vi "IF2_TagDataConversion.vi"(8 "error in (no error)":errorcluster, 10 "IF2 Data":string, 11 "TCP Network Connection in":refnum<k5>) -> (0 "error out":errorcluster, 3 "TCP Network Connection out":refnum<k5>)   [LabVIEW 2015, in "IF2_Reader.lvlib"]
uses:
  IF2_Reader.lvlib
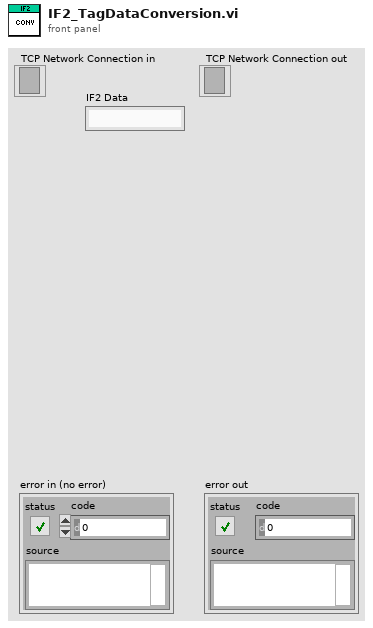
[diagram p1: front panel]
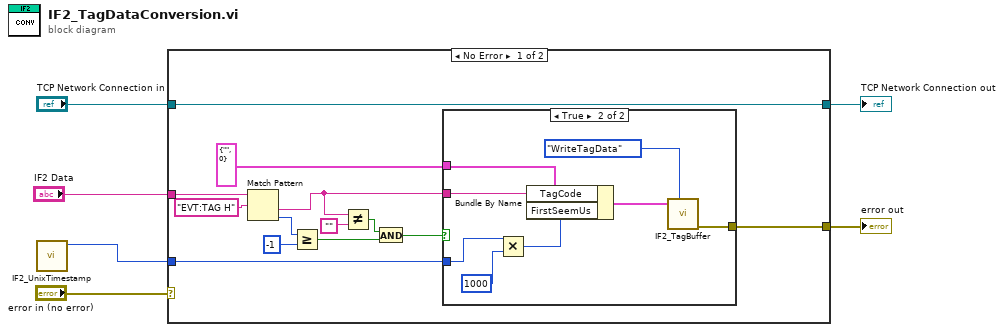
[diagram p0: block diagram]
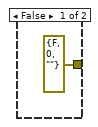
[diagram p2: hidden frame]
diagram:
  n1 = call "IF2_UnixTimestamp.vi"() -> ("unixTimeStamp"=w1:u64)  [unwired: 11 in]
  n2 = case shown="No Error" "error in (no error)" {
    selector: "error in (no error)" -> [_ w29]
    tunnel: "TCP Network Connection in" -> [w16 w30]
    tunnel: [w16 w30] -> w4
    tunnel: [w18 w29] -> w6
    tunnel: "IF2 Data" -> [w14 _]
    tunnel: w1 -> [w15 _]
    frame No Error {
      n3 = Match Pattern(string=w14, regular expression="EVT:TAG H") -> (after substring=w9:string, offset past match=w13:i32)  [unwired: 3 out]
      n4 = Greater Or Equal?(x=w13, y=-1) -> (x >= y?=w11:bool)
      n5 = Not Equal?(x=w9, y="") -> (x != y?=w7:bool)
      n6 = And(x=w7, y=w11) -> (x .and. y?=w10:bool)
      n7 = case shown="True" w10 {
        tunnel: [errorcluster {"status"=FALSE, "code"=0, "source"=""} ("error out") w23] -> w18
        tunnel: w9 -> [_ w27]
        tunnel: cluster{"TagCode":string, "FirstSeemUs":u64} {"TagCode"="", "FirstSeemUs"=0} ("TagData in") -> [_ w28]
        tunnel: w15 -> [_ w26]
        frame False {
        }
        frame True {
          n8 = Multiply(x=w26, y=u64 1000) -> (x*y=w21:u64)
          n9 = Bundle By Name(cluster=w28, "TagCode"=w27, "FirstSeemUs"=w21) -> (w24:cluster{"TagCode":string, "FirstSeemUs":u64})
          n10 = call "IF2_TagBuffer.vi"("Action"=enum16{"Init", "WriteTagData", "ReadTagData"}."WriteTagData", "TagData in"=w24) -> ("error out"=w23:errorcluster)  [unwired: 8 in, 1 out]
        }
      }
    }
    frame Error {
    }
  }
  "TCP Network Connection out" <- w4
  "error out" <- w6
